vi "Sin Cos.vi"(11 "Angle":dbl) -> (2 "Cos":dbl, 3 "Sin":dbl)   [LabVIEW 2020]
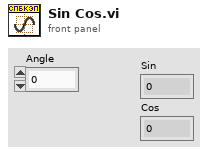
[diagram p1: front panel]
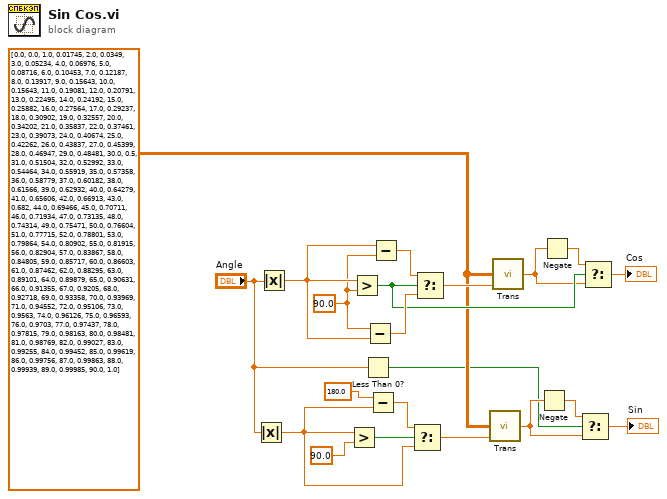
[diagram p0: block diagram]
diagram:
  w18 = 90.0 ("y")
  w6 = dbl[][] [[0.0, 0.0], [1.0, 0.01745], [2.0, 0.0349], [3.0, 0.05234], [4.0, 0.06976], [5.0, 0.08716], [6.0, 0.10453], [7.0, 0.12187], [8.0, 0.13917], [9.0, 0.15643], [10.0, 0.15643], [11.0, 0.19081], [12.0, 0.20791], [13.0, 0.22495], [14.0, 0.24192], [15.0, 0.25882], [16.0, 0.27564], [17.0, 0.29237], [18.0, 0.30902], [19.0, 0.32557], [20.0, 0.34202], [21.0, 0.35837], [22.0, 0.37461], [23.0, 0.39073], [24.0, 0.40674], [25.0, 0.42262], [26.0, 0.43837], [27.0, 0.45399], [28.0, 0.46947], [29.0, 0.48481], [30.0, 0.5], [31.0, 0.51504], [32.0, 0.52992], [33.0, 0.54464], [34.0, 0.55919], [35.0, 0.57358], [36.0, 0.58779], [37.0, 0.60182], [38.0, 0.61566], [39.0, 0.62932], [40.0, 0.64279], [41.0, 0.65606], [42.0, 0.66913], [43.0, 0.682], [44.0, 0.69466], [45.0, 0.70711], [46.0, 0.71934], [47.0, 0.73135], [48.0, 0.74314], [49.0, 0.75471], [50.0, 0.76604], [51.0, 0.77715], [52.0, 0.78801], [53.0, 0.79864], [54.0, 0.80902], [55.0, 0.81915], [56.0, 0.82904], [57.0, 0.83867], [58.0, 0.84805], [59.0, 0.85717], [60.0, 0.86603], [61.0, 0.87462], [62.0, 0.88295], [63.0, 0.89101], [64.0, 0.89879], [65.0, 0.90631], [66.0, 0.91355], [67.0, 0.9205], [68.0, 0.92718], [69.0, 0.93358], [70.0, 0.93969], [71.0, 0.94552], [72.0, 0.95106], [73.0, 0.9563], [74.0, 0.96126], [75.0, 0.96593], [76.0, 0.9703], [77.0, 0.97437], [78.0, 0.97815], [79.0, 0.98163], [80.0, 0.98481], [81.0, 0.98769], [82.0, 0.99027], [83.0, 0.99255], [84.0, 0.99452], [85.0, 0.99619], [86.0, 0.99756], [87.0, 0.99863], [88.0, 0.99939], [89.0, 0.99985], [90.0, 1.0]] ("Array 4")
  n1 = Absolute Value(x="Angle") -> (abs(x)=w5:dbl)
  n2 = Absolute Value(x="Angle") -> (abs(x)=w19:dbl)
  n3 = Greater?(x=w5, y=90.0) -> (0:w10:bool)
  n4 = Greater?(x=w19, y=w18) -> (0:w15:bool)
  n5 = Less Than 0?(x="Angle") -> (x < 0?=w2:bool)
  n6 = Subtract(x=w18, y=w19) -> (x-y=w21:dbl)
  n7 = Subtract(x=180.0, y=w5) -> (x-y=w7:dbl)
  n8 = Subtract(x=w19, y=w18) -> (x-y=w20:dbl)
  n9 = Select(t=w7, s=w10, f=w5) -> (s? t:f=w9:dbl)
  n10 = Select(t=w20, s=w15, f=w21) -> (s? t:f=w17:dbl)
  n11 = call "Trans.vi"("Y"=w9, "Array 4"=w6) -> ("Y value"=w12:dbl)  [unwired: 1 in]
  n12 = call "Trans.vi"("Y"=w17, "Array 4"=w6) -> ("Y value"=w13:dbl)  [unwired: 1 in]
  n13 = Negate(x=w12) -> (-x=w11:dbl)
  n14 = Negate(x=w13) -> (-x=w14:dbl)
  n15 = Select(t=w11, s=w2, f=w12) -> (s? t:f=→"Sin":dbl)
  n16 = Select(t=w14, s=w15, f=w13) -> (s? t:f=→"Cos":dbl)
